vi "Display Annotation.vi"(0 "VISA resource name":refnum<visa-resource-name>, 5 "Display Window Annotation (T:Enable)":bool=TRUE, 11 "error in (no error)":errorcluster) -> (4 "VISA resource name out":refnum<visa-resource-name>, 15 "error out":errorcluster)   [LabVIEW 2020, in "Anritsu Signal Analyzer Series.lvlib"]
doc: "Turns On/Off Display Annotation. When set to Off, the frequency and level of the measurement target are hidden from the screen."
uses:
  Anritsu Signal Analyzer Series.lvlib
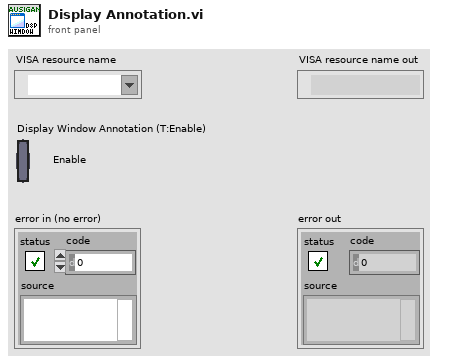
[diagram p1: front panel]
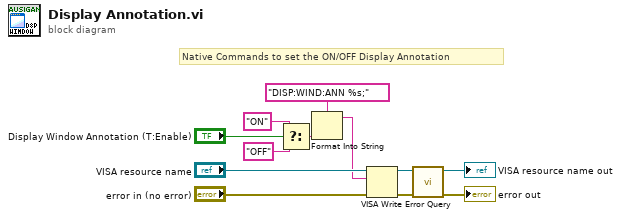
[diagram p0: block diagram]
diagram:
  # "Native Commands to set the ON/OFF Display Annotation"
  n1 = Select(t="ON", s="Display Window Annotation (T:Enable)", f="OFF") -> (s? t:f=w4:string)
  n2 = Format Into String(format string="DISP:WIND:ANN %s;" ("_CommandSet"), w4) -> (resulting string=w1:string)  [unwired: 2 in, 1 out]
  n3 = VISA Write(VISA resource name="VISA resource name", write buffer=w1, error in (no error)="error in (no error)") -> (VISA resource name out=w10:refnum<visa-resource-name>, error out=w9:errorcluster)  [unwired: 1 out]
  n4 = call "Error Query.vi"("error in (no error)"=w9, "VISA resource name"=w10) -> ("error out"=→"error out":errorcluster, "VISA resource name out"=→"VISA resource name out":refnum<visa-resource-name>)  [unwired: 6 in, 2 out]
